vi "XY data formatting.vi"(8 "error in (no error)":errorcluster, 11 "App Data":T1) -> (0 "error out":errorcluster, 3 "Array":T2(array[cluster]))   [LabVIEW 2014]
uses:
  Controls/App Data.ctl
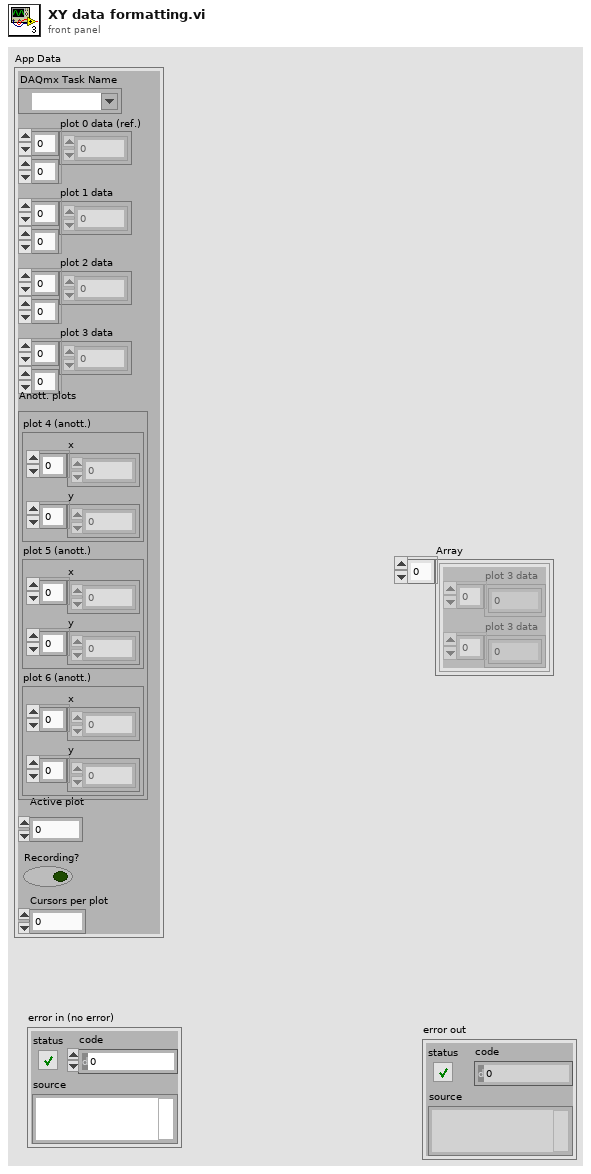
[diagram p1: front panel]
types:
  T1 = typedef "App Data.ctl" = cluster{"DAQmx Task Name":refnum<k21>, "plot 0 data (ref.)":dbl[][], "plot 1 data":dbl[][], "plot 2 data":dbl[][], "plot 3 data":dbl[][], "Anott. plots":cluster{"plot 4 (anott.)":cluster{"x":dbl[], "y":dbl[]}, "plot 5 (anott.)":cluster{"x":dbl[], "y":dbl[]}, "plot 6 (anott.)":cluster{"x":dbl[], "y":dbl[]}}, "Active plot":u32, "Recording?":bool, "Cursors per plot":i32}
  T2 = cluster{"plot 3 data":dbl[], "plot 3 data":dbl[]}[]
  T3 = cluster{"plot 4 (anott.)":cluster{"x":dbl[], "y":dbl[]}, "plot 5 (anott.)":cluster{"x":dbl[], "y":dbl[]}, "plot 6 (anott.)":cluster{"x":dbl[], "y":dbl[]}}
  T4 = cluster{"plot 0 data (ref.)":dbl[], "plot 0 data (ref.)":dbl[]}
  T5 = cluster{"plot 3 data":dbl[], "plot 3 data":dbl[]}
  T6 = cluster{"plot 1 data":dbl[], "plot 1 data":dbl[]}
  T7 = cluster{"plot 2 data":dbl[], "plot 2 data":dbl[]}
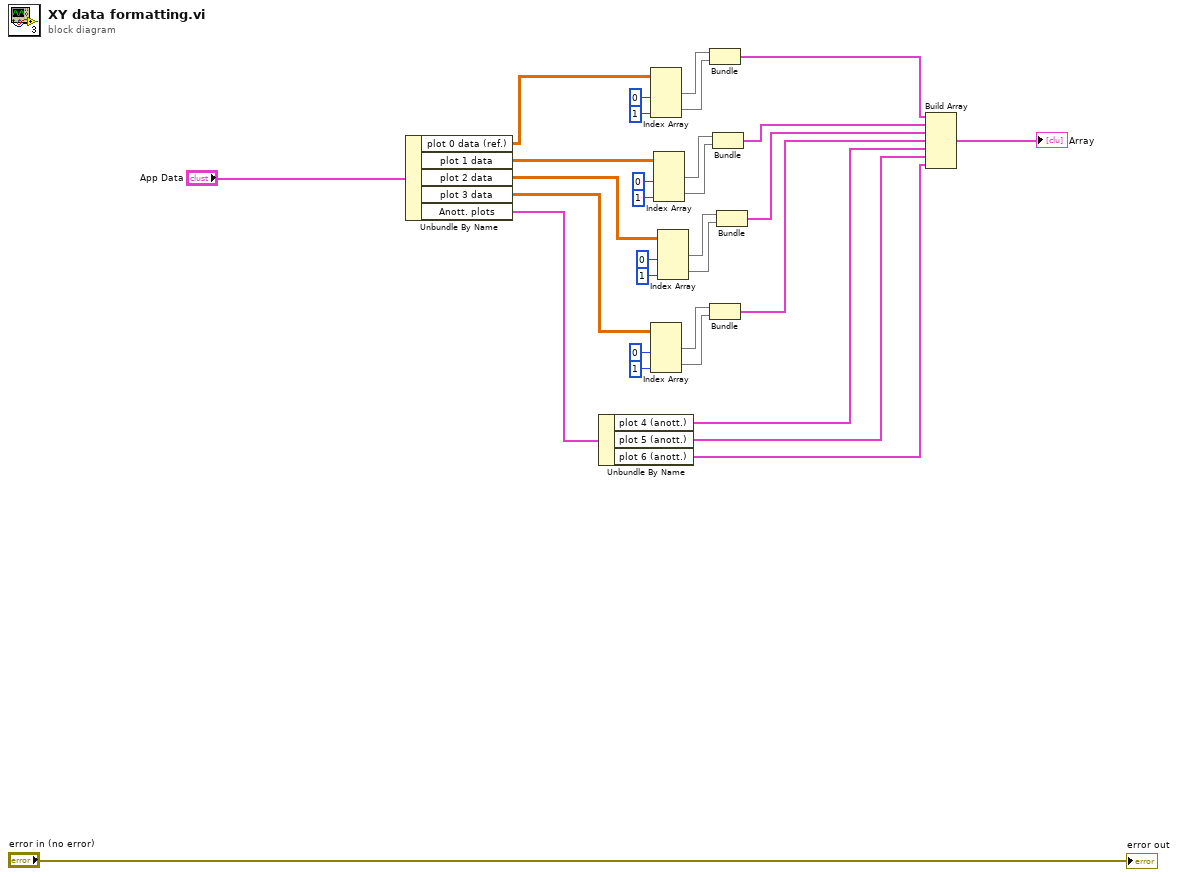
[diagram p0: block diagram]
diagram:
  n1 = Unbundle By Name("App Data") -> ("plot 0 data (ref.)"=w6:dbl[][], "plot 1 data"=w13:dbl[][], "plot 2 data"=w29:dbl[][], "plot 3 data"=w30:dbl[][], "Anott. plots"=w1:T3)
  n2 = Unbundle By Name(w1) -> ("plot 4 (anott.)"=w4:cluster{"x":dbl[], "y":dbl[]}, "plot 5 (anott.)"=w3:cluster{"x":dbl[], "y":dbl[]}, "plot 6 (anott.)"=w2:cluster{"x":dbl[], "y":dbl[]})
  n3 = Index Array(array=w6, index (col) #1=0 ("disabled index (col)"), index (col) #2=1 ("index (col)")) -> (element #1=w9:dbl[], element #2=w10:dbl[])  [unwired: 2 in]
  n4 = Index Array(array=w30, index (col) #1=0 ("disabled index (col)"), index (col) #2=1 ("index (col)")) -> (element #1=w26:dbl[], element #2=w27:dbl[])  [unwired: 2 in]
  n5 = Index Array(array=w13, index (col) #1=0 ("disabled index (col)"), index (col) #2=1 ("index (col)")) -> (element #1=w16:dbl[], element #2=w17:dbl[])  [unwired: 2 in]
  n6 = Index Array(array=w29, index (col) #1=0 ("disabled index (col)"), index (col) #2=1 ("index (col)")) -> (element #1=w21:dbl[], element #2=w20:dbl[])  [unwired: 2 in]
  n7 = Bundle("plot 0 data (ref.)"=w9, "plot 0 data (ref.)"=w10) -> (w5:T4)  [unwired: 1 in]
  n8 = Bundle("plot 3 data"=w26, "plot 3 data"=w27) -> (w31:T5)  [unwired: 1 in]
  n9 = Bundle("plot 1 data"=w16, "plot 1 data"=w17) -> (w19:T6)  [unwired: 1 in]
  n10 = Bundle("plot 2 data"=w21, "plot 2 data"=w20) -> (w28:T7)  [unwired: 1 in]
  n11 = Build Array(w5, w19, w28, w31, w4, w3, w2) -> (→"Array":cluster{"x":dbl[], "y":dbl[]}[])
  "error out" <- "error in (no error)"
